vi "Remote Client.vi"(6 "Wait for Response? [T]":bool=TRUE, 8 "error in (no error)":errorcluster, 9 "Data":variant, 10 "Command":string, 11 "Instrument in":refnum<class "Instrument.lvclass">) -> (0 "error out":errorcluster, 1 "Data out":variant, 2 "Command out":string, 3 "Instrument out":refnum<class "Instrument.lvclass">)   [LabVIEW 2016, in "Instrument.lvclass"]
uses:
  Instrument.lvclass
  <userlib>/_OpenG.lib/numeric/numeric.llb/Random Number Within Range - I32__ogtk.vi
  RemoteControl/RemoteControl.lvclass
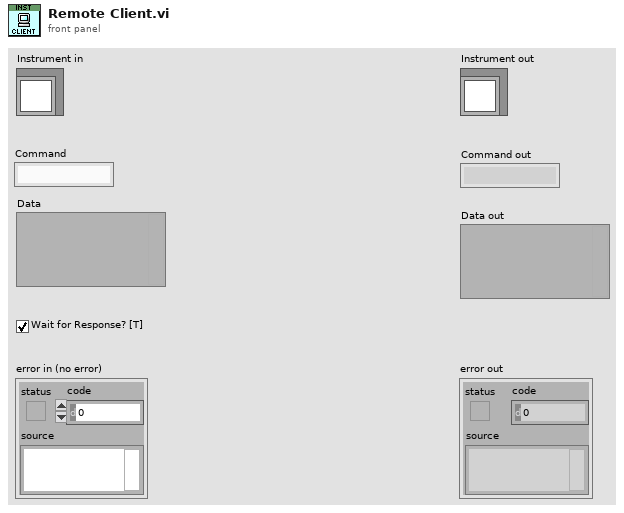
[diagram p1: front panel]
types:
  T1 = typedef "Instrument.lvclass/PublicEvents--Cluster.ctl" = cluster{"MessageFromProcess":refnum<user-event>}
  T2 = typedef "Instrument.lvclass/SMO RC Type--enum.ctl" = enum16{"RC", "STM", "ZMQ"}
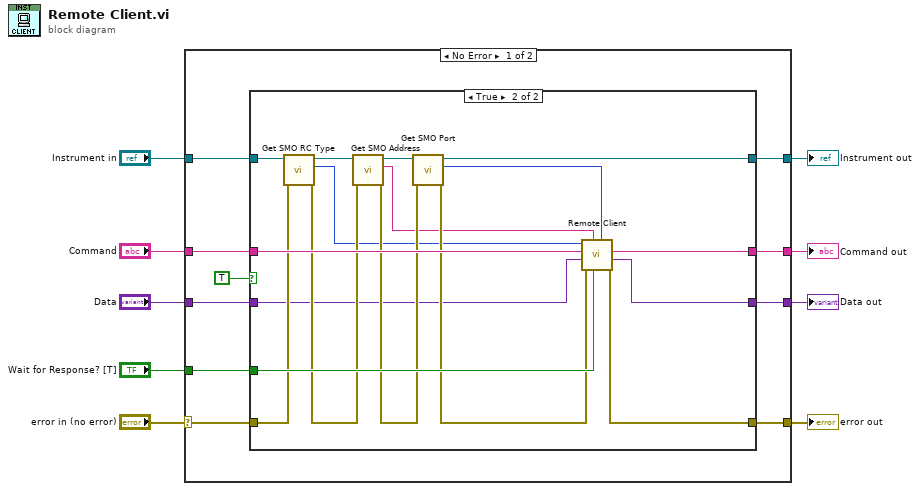
[diagram p0: block diagram]
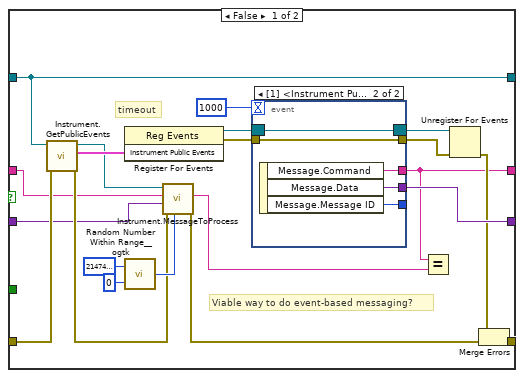
[diagram p2: hidden frame]
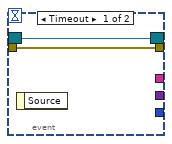
[diagram p3: hidden frame]
diagram:
  n1 = case shown="No Error" "error in (no error)" {
    selector: "error in (no error)" -> [w19 w66]
    tunnel: [w18 w66] -> w8
    tunnel: [w10 w65] -> w6
    tunnel: "Instrument in" -> [w11 w65]
    tunnel: [w17 _] -> w5
    tunnel: [w13 w64] -> w4
    tunnel: "Command" -> [w14 w64]
    tunnel: "Data" -> [w16 _]
    tunnel: "Wait for Response? [T]" -> [w15 _]
    frame No Error {
      n2 = case shown="True" TRUE {
        tunnel: w19 -> [w30 w57]
        tunnel: [w26 w63] -> w18
        tunnel: [w35 w47] -> w17
        tunnel: w16 -> [w20 w48]
        tunnel: w15 -> [_ w62]
        tunnel: w11 -> [w24 w59]
        tunnel: w14 -> [w21 w60]
        tunnel: [w22 w61] -> w13
        tunnel: [w24 w58] -> w10
        frame False {
          # "Viable way to do event-based messaging?"
          # "timeout"
          n3 = call "Instrument.GetPublicEvents.vi"("error in (no error)"=w30, "Instrument"=w24) -> ("error out"=w29:errorcluster, "Instrument Public Events"=w37:T1, "Instrument out"=w23:refnum<class "Instrument.lvclass">)  [unwired: 7 in]
          n4 = register-events(w37) -> (reference out=w36:refnum<event-registration>, error out=w32:errorcluster)  [unwired: 2 in]
          n5 = call-poly <userlib>:"Random Number Within Range__ogtk.vi"("High"=2147483647, "Low"=0) -> ("Random Number"=w31:i32)  [unwired: 3 in]
          n6 = call "Instrument.MessageToProcess.vi"("Message ID"=w31, "error in (no error)"=w29, "Message.Data"=w20, "Message.Command"=w21, "Instrument"=w23) -> ("error out"=w25:errorcluster)  [unwired: 5 in, 1 out]
          n7 = event shown="[1] <Instrument Public Events.MessageFromProcess>: User Event" {
            selector: w36 -> [w40 w42]
            dyn-events: [w40 w42] -> w28
            timeout: 1000 -> [_ _]
            tunnel: [_ w46] -> w22
            tunnel: [_ w45] -> w35
            tunnel: [w41 w44] -> w33
            tunnel: w32 -> [w41 w44]
            tunnel: [_ w43] -> _
            event Timeout {
              n8 = event-data() -> ()  [unwired: 1 in, 1 out]
            }
            event User Event {
              n9 = event-data() -> ("Message.Command"=w46:string, "Message.Data"=w45:variant, "Message.Message ID"=w43:i32)  [unwired: 1 in]
            }
          }
          n10 = Equal?(x=w22, y=w21) -> ()  [unwired: 1 out]
          n11 = Unregister For Events(event registration refnum=w28, error in=w33) -> (error out=w27:errorcluster)
          n12 = Merge Errors(w27, w25) -> (w26:errorcluster)
        }
        frame True {
          n13 = call-dynamic "Get SMO RC Type.vi"("error in (no error)"=w57, "Instrument in"=w59) -> ("error out"=w53:errorcluster, "RC Type"=w51:T2, "Instrument out"=w55:refnum<class "Instrument.lvclass">)  [unwired: 7 in]
          n14 = call-dynamic "Get SMO Address.vi"("error in (no error)"=w53, "Instrument in"=w55) -> ("error out"=w52:errorcluster, "SMO Address"=w50:string, "Instrument out"=w54:refnum<class "Instrument.lvclass">)  [unwired: 7 in]
          n15 = call-dynamic "Get SMO Port.vi"("error in (no error)"=w52, "Instrument in"=w54) -> ("error out"=w56:errorcluster, "Port"=w49:u16, "Instrument out"=w58:refnum<class "Instrument.lvclass">)  [unwired: 7 in]
          n16 = call "Remote Client.vi"("Port"=w49, "Wait for Response?"=w62, "address"=w50, "error in (no error)"=w56, "Data"=w48, "Command"=w60, "RC Type"=w51) -> ("error out"=w63:errorcluster, "Data out"=w47:variant, "Command out"=w61:string)  [unwired: 1 in, 1 out]
        }
      }
    }
    frame Error {
    }
  }
  "error out" <- w8
  "Instrument out" <- w6
  "Command out" <- w4
  "Data out" <- w5
